vi "exRampTriangleGenerator.vi"(1 "Number of positions":u16, 2 "End(um)":dbl, 3 "Start(um)":dbl) -> (0 "Array":dbl[](array[numeric]))   [LabVIEW 2026]
panel:
  out "step size":dbl
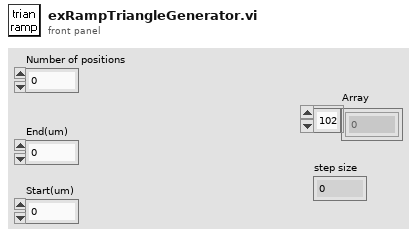
[diagram p1: front panel]
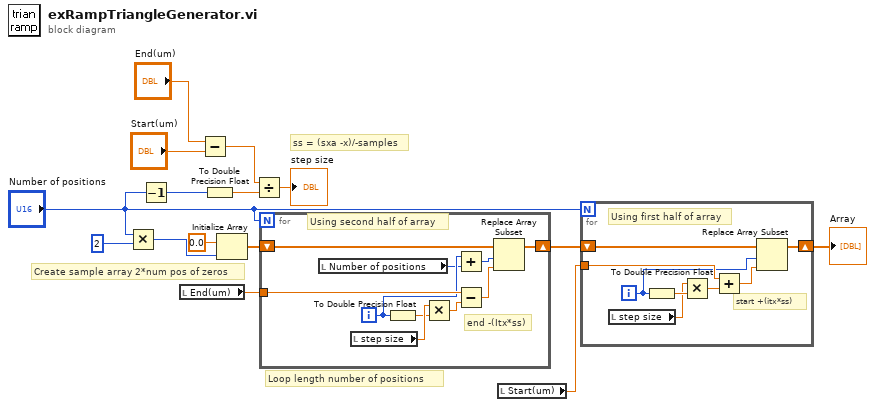
[diagram p0: block diagram]
diagram:
  # "Loop length number of positions"
  # "Create sample array 2*num pos of zeros"
  # "ss = (sxa -x)/-samples"
  n1 = Multiply(x="Number of positions", y=u16 2) -> (x*y=w8:u16)
  n2 = Decrement(x="Number of positions") -> (x-1=w11:u16)
  n3 = local read "End(um)"() -> (w3:dbl)
  n4 = Subtract(x="End(um)", y="Start(um)") -> (x-y=w13:dbl)
  n5 = To Double Precision Float(number=w11) -> (double precision float=w10:dbl)
  n6 = Initialize Array(0.0, w8) -> (w7:dbl[])
  n7 = Divide(x=w13, y=w10) -> (x/y=→"step size":dbl)
  n8 = for {
    N: "Number of positions" -> [_]
    shift-right: [w24] -> w6
    shift-left: w7 -> [w25]
    tunnel: w3 -> [w23]
    i -> [w18]
    # "end -(Itx*ss)"
    # "Using second half of array"
    n9 = local read "Number of positions"() -> (w16:u16)
    n10 = local read "step size"() -> (w21:dbl)
    n11 = To Double Precision Float(number=w18) -> (double precision float=w20:dbl)
    n12 = Multiply(x=w21, y=w20) -> (x*y=w19:dbl)
    n13 = Add(x=w18, y=w16) -> (x+y=w17:i32)
    n14 = Subtract(x=w23, y=w19) -> (x-y=w22:dbl)
    n15 = Replace Array Subset(array=w25, new element=w22, index=w17) -> (w24:dbl[])
  }
  n16 = local read "Start(um)"() -> (w5:dbl)
  n17 = for {
    N: "Number of positions" -> [_]
    tunnel: w5 -> [w32]
    shift-right: [w27] -> w1
    shift-left: w6 -> [w28]
    i -> [w30]
    # "start +(itx*ss)"
    # "Using first half of array"
    n18 = local read "step size"() -> (w26:dbl)
    n19 = To Double Precision Float(number=w30) -> (double precision float=w29:dbl)
    n20 = Multiply(x=w26, y=w29) -> (x*y=w33:dbl)
    n21 = Add(x=w32, y=w33) -> (x+y=w31:dbl)
    n22 = Replace Array Subset(array=w28, new element=w31, index=w30) -> (w27:dbl[])
  }
  "Array" <- w1
